vi "Databases.vi"(8 "error in (no error)":errorcluster, 11 "Node Ptr":T1 format="%.0x") -> (0 "error out":errorcluster)   [LabVIEW 2020, in "AIM ARINC 664 System Explorer.lvlib" / "Implementation.lvlib"]
uses:
  Implementation.lvlib
  <vilib>/NI VeriStand/Custom Device API/Custom Device API.lvlib
  <vilib>/NI VeriStand/Custom Device API/Custom Device Item Ref.ctl
panel:
  in  "SHDocVw.IWebBrowser":refnum<k7>(container)
  in  "Specific Header":cluster{"Section Name":string}={"Section Name"="Specific Page Settings"}
  in  "General Header":cluster{"Section Name":string}={"Section Name"="General Page Settings"}
  in  "Description":string
  in  "Name":string
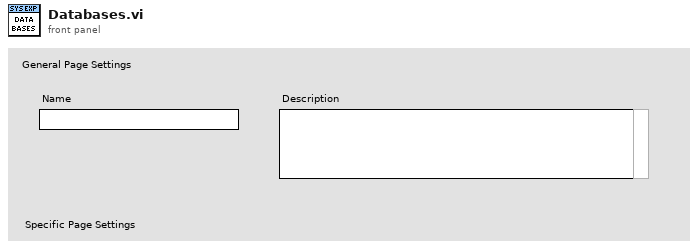
[diagram p1: front panel]
types:
  T1 = typedef "Custom Device API.lvlib/Custom Device Item Ref.ctl" = u64
  T2 = typedef "Custom Device API.lvlib/Custom Device Item Info.ctl" = cluster{"Name":string, "Is Channel":bool, "GUID":string, "Is Waveform":bool}
  T3 = typedef "Custom Device API.lvlib/Custom Device Commands.ctl" = enum16{"Default", "Item renamed", "Shutdown", "Dynamic button pressed"}
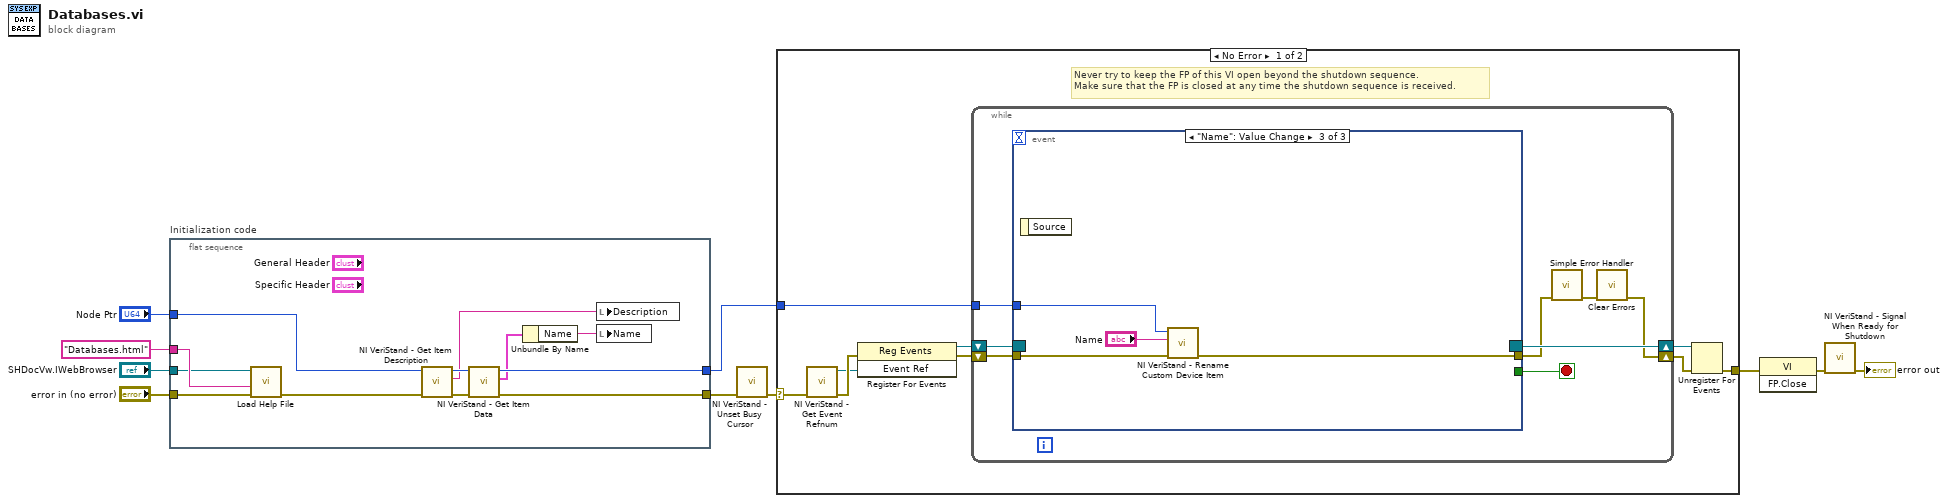
[diagram p0: block diagram]
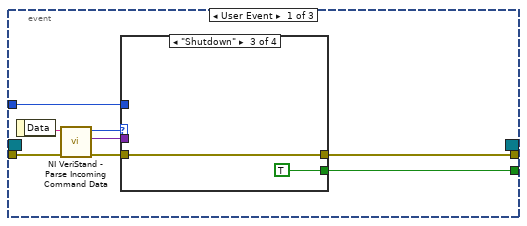
[diagram p2: hidden frame]
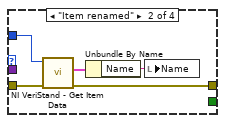
[diagram p4: hidden frame]
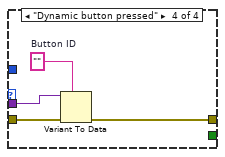
[diagram p5: hidden frame]
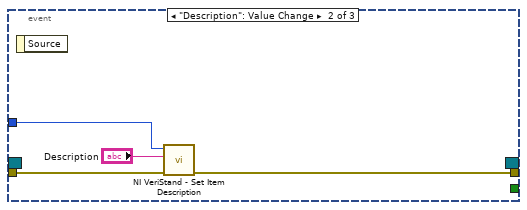
[diagram p6: hidden frame]
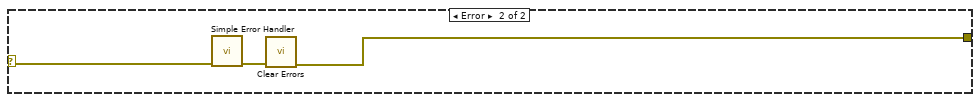
[diagram p7: hidden frame]
diagram:
  n1 = flat-sequence "Initialization code" {
    tunnel: "error in (no error)" -> [w15]
    tunnel: "Node Ptr" -> [w17]
    tunnel: [w18] -> w6
    tunnel: [w22] -> w3
    tunnel: "SHDocVw.IWebBrowser" -> [w12]
    tunnel: "Databases.html" ("CD_CHM_Section") -> [w13]
    frame #0 {
      n2 = call "Load Help File.vi"("error in (no error)"=w15, "HTML File to Load"=w13, "Browser"=w12) -> ("error out"=w14:errorcluster)  [unwired: 8 in]
      n3 = call <vilib>:"NI VeriStand - Get Item Description.vi"("error in (no error)"=w14, "Item Ref in"=w17) -> ("error out"=w20:errorcluster, "Description"=w16:string, "Item Ref out"=w21:T1)  [unwired: 7 out]
      n4 = call <vilib>:"NI VeriStand - Get Item Data.vi"("error in (no error)"=w20, "Item Ref in"=w21) -> ("error out"=w18:errorcluster, "Item Info"=w19:T2, "Item Ref out"=w22:T1)  [unwired: 7 out]
      n5 = Unbundle By Name(w19) -> ("Name"=w11:string)
      n6 = local write "Description"(w16) -> ()
      n7 = local write "Name"(w11) -> ()
    }
  }
  n8 = call <vilib>:"NI VeriStand - Unset Busy Cursor.vi"("error in (no error)"=w6) -> ("error out"=w5:errorcluster)  [unwired: 10 out]
  n9 = case shown="No Error" w5 {
    selector: w5 -> [w23 w70]
    tunnel: [w28 w68] -> w10
    tunnel: w3 -> [w24 _]
    frame No Error {
      # "Never try to keep the FP of this VI open beyond the shutdown sequence.\nMake sure that the FP is closed at any time the shutdown sequence is received."
      n10 = call <vilib>:"NI VeriStand - Get Event Refnum.vi"("error in (no error)"=w23) -> ("error out"=w31:errorcluster, "Event Ref"=w27:refnum<user-event>)  [unwired: 9 out]
      n11 = register-events(error in=w31, w27) -> (reference out=w25:refnum<event-registration>, error out=w26:errorcluster)  [unwired: 1 in]
      n12 = while {
        tunnel: w24 -> [w35]
        shift-right: [w32] -> w29
        shift-left: w26 -> [w38]
        shift-right: [w39] -> w30
        shift-left: w25 -> [w37]
        stop <- w36 stop-if-true
        n13 = event shown="[2] \"Name\": Value Change" {
          selector: w37 -> [_ _ _]
          dyn-events: [_ _ _] -> w39
          timeout: _ -> [_ _ _]
          tunnel: w38 -> [w47 w62 w66]
          tunnel: [w43 _ _] -> w36
          tunnel: [w42 w61 w65] -> w34
          tunnel: w35 -> [w41 w63 w67]
          event User Event {
            n14 = event-data() -> ("Data"=w46:string)  [unwired: 1 out]
            n15 = call <vilib>:"NI VeriStand - Parse Incoming Command Data.vi"("error in (no error)"=w47, "Incoming data"=w46) -> ("error out"=w45:errorcluster, "Outgoing data"=w40:variant, "Action"=w44:T3)  [unwired: 7 out]
            n16 = case shown="\"Shutdown\"" w44 {
              tunnel: w45 -> [w48 w53 w54 w59]
              tunnel: [_ _ TRUE _] -> w43
              tunnel: [w48 w50 w54 w56] -> w42
              tunnel: w41 -> [_ w52 _ _]
              tunnel: w40 -> [_ _ _ w58]
              frame "Default", Default {
              }
              frame "Item renamed" {
                n17 = call <vilib>:"NI VeriStand - Get Item Data.vi"("error in (no error)"=w53, "Item Ref in"=w52) -> ("error out"=w50:errorcluster, "Item Info"=w51:T2)  [unwired: 8 out]
                n18 = Unbundle By Name(w51) -> ("Name"=w49:string)
                n19 = local write "Name"(w49) -> ()
              }
              frame "Shutdown" {
              }
              frame "Dynamic button pressed" {
                w57 = ""  # Button ID
                n20 = Variant To Data(error in=w59, type=w57, Variant=w58) -> (error out=w56:errorcluster)  [unwired: 1 out]
              }
            }
          }
          event "Description": Value Change {
            n21 = event-data() -> ()  [unwired: 2 out]
            n22 = call <vilib>:"NI VeriStand - Set Item Description.vi"("error in (no error)"=w62, "Description"="Description", "Item Ref in"=w63) -> ("error out"=w61:errorcluster)  [unwired: 8 out]
          }
          event "Name": Value Change {
            n23 = event-data() -> ()  [unwired: 2 out]
            n24 = call <vilib>:"NI VeriStand - Rename Custom Device Item.vi"("error in (no error)"=w66, "New Name"="Name", "Item Ref in"=w67) -> ("error out"=w65:errorcluster)  [unwired: 6 in, 2 out]
          }
        }
        n25 = call <vilib>:"Simple Error Handler.vi"("error in (no error)"=w34) -> ("error out"=w33:errorcluster)  [unwired: 1 in, 7 out]
        n26 = call <vilib>:"Clear Errors.vi"("error in (no error)"=w33) -> ("error out"=w32:errorcluster)  [unwired: 1 in, 5 out]
      }
      n27 = Unregister For Events(event registration refnum=w30, error in=w29) -> (error out=w28:errorcluster)
    }
    frame Error {
      n28 = call <vilib>:"Simple Error Handler.vi"("error in (no error)"=w70) -> ("error out"=w69:errorcluster)  [unwired: 1 in, 7 out]
      n29 = call <vilib>:"Clear Errors.vi"("error in (no error)"=w69) -> ("error out"=w68:errorcluster)  [unwired: 1 in, 5 out]
    }
  }
  n30 = invoke class="VI" method="FP.Close"(error in=w10) -> (error out=w9:errorcluster)  [unwired: 2 in, 2 out]
  n31 = call <vilib>:"NI VeriStand - Signal When Ready for Shutdown.vi"("error in (no error)"=w9) -> ("error out"=→"error out":errorcluster)  [unwired: 10 out]
